vi "All parameter error estimate.vi"(8 "covariance":T2, 9 "best fit parameters":dbl[](array[numeric]), 10 "best nonlinear fit":dbl[](array[numeric]), 11 "Y":dbl[](array[numeric])) -> (0 "Status":i32[](array[numeric]), 1 "R-square":dbl, 2 "All FWHM":dbl[](array[numeric]), 3 "All Parameters Fit":T1(array[cluster]), 4 "List Status":string[][](table))   [LabVIEW 2023]
uses:
  <vilib>/Analysis/Matrix/Datatypes/RealMatrix.ctl
  <vilib>/Analysis/Matrix/Numeric/Conversions/Array To Matrix - RA2.vi
  <vilib>/Analysis/NI_AALPro.lvlib
  <vilib>/Analysis/Matrix/NI_Matrix.lvlib
panel:
  out "Correlation Matrix":T2
  out "Parameters Fit":T3
  out "FWHM":dbl
  out "Error":dbl[](array[numeric])
  out "RMSE":dbl
  out "SSE":dbl
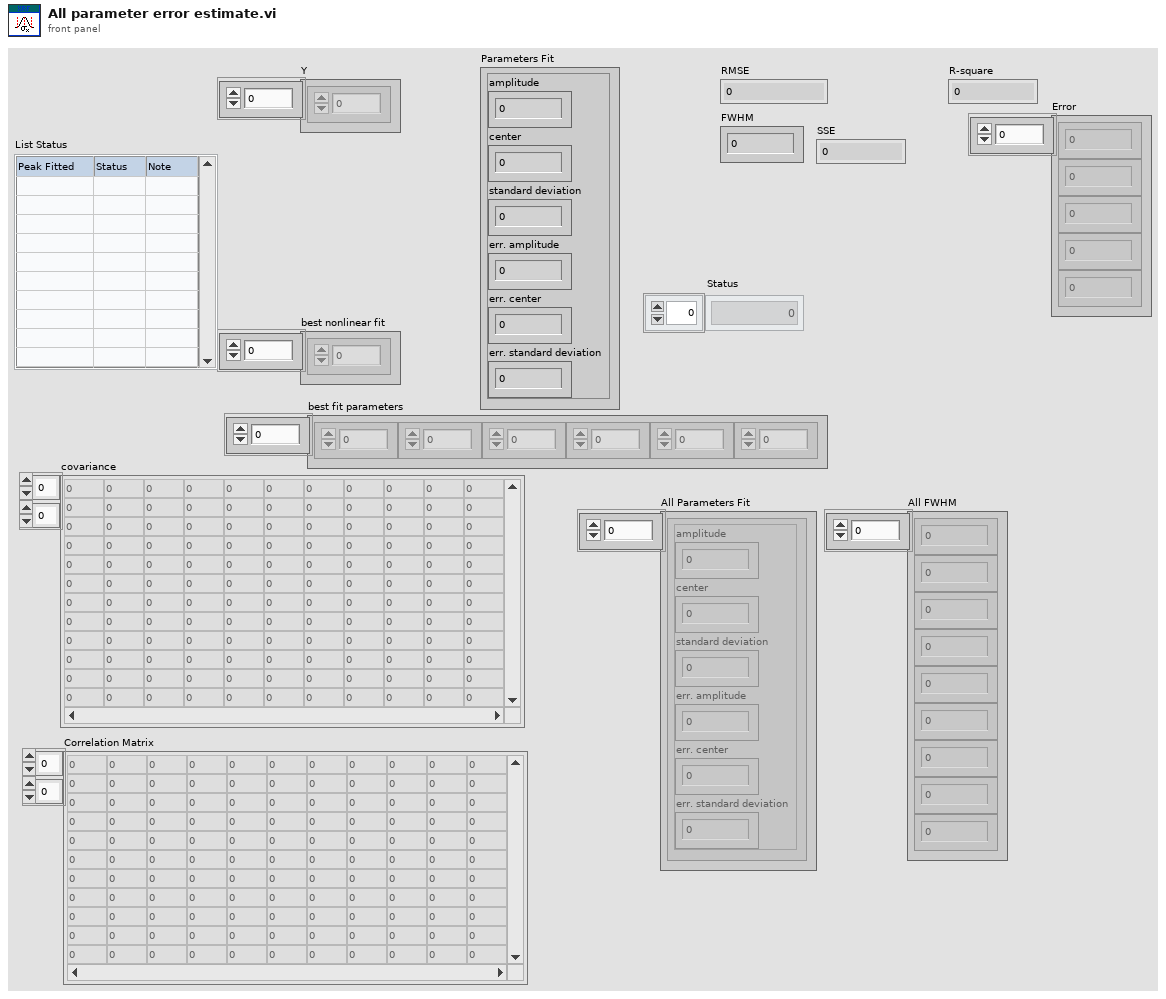
[diagram p1: front panel]
types:
  T1 = cluster{"amplitude":dbl, "center":dbl, "standard deviation":dbl, "err. amplitude":dbl, "err. center":dbl, "err. standard deviation":dbl}[]
  T2 = typedef "NI_Matrix.lvlib/RealMatrix.ctl" = dbl[][]
  T3 = cluster{"amplitude":dbl, "center":dbl, "standard deviation":dbl, "err. amplitude":dbl, "err. center":dbl, "err. standard deviation":dbl}
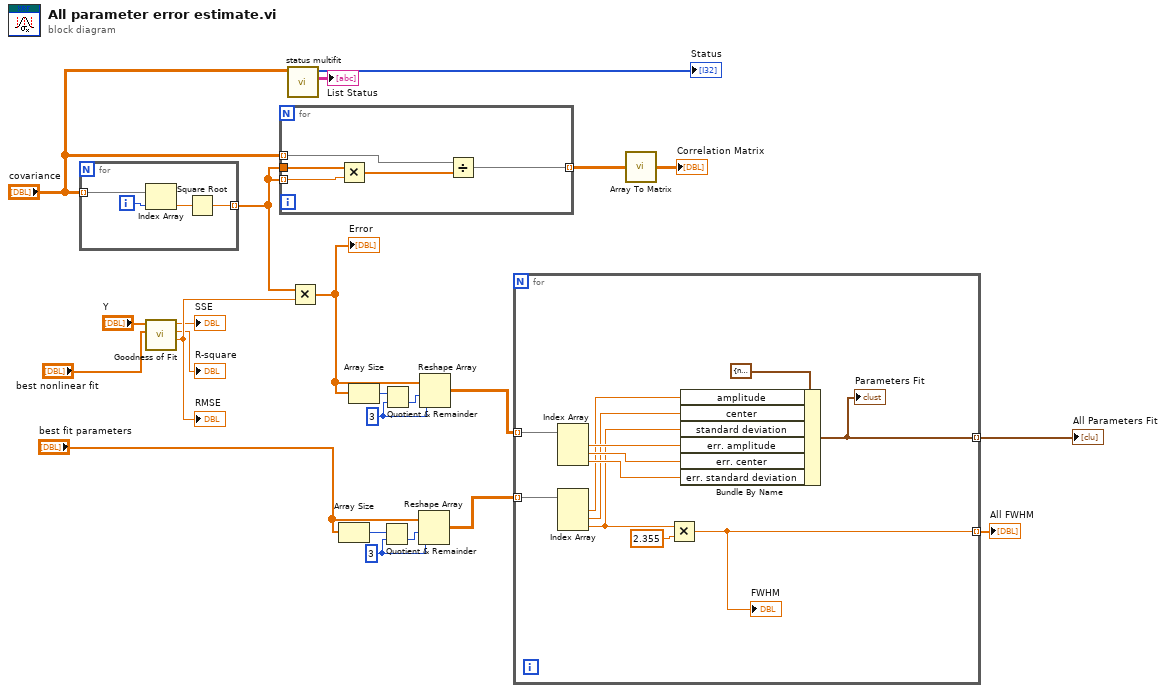
[diagram p0: block diagram]
diagram:
  w13 = 3 ("y")
  w14 = 3 ("y")
  n1 = for {
    tunnel: "covariance" -> [w27] mode=indexing
    tunnel: [w24] -> w19 mode=indexing
    i -> [w26]
    n2 = Index Array(array=w27, index=w26) -> (element=w25:dbl)
    n3 = Square Root(x=w25) -> (sqrt(x)=w24:dbl)
  }
  n4 = call <vilib>:"Goodness of Fit.vi"("Best Fit"="best nonlinear fit", "Y"="Y") -> ("RMSE"=w23:dbl, "R-square"=→"R-square":dbl, "SSE"=→"SSE":dbl)  [unwired: 6 in, 1 out]
  "RMSE" <- w23
  n5 = for {
    tunnel: "covariance" -> [w29] mode=indexing
    tunnel: w19 -> [w31]
    tunnel: w19 -> [w32] mode=indexing
    tunnel: [w28] -> w20 mode=indexing
    n6 = Multiply(x=w31, y=w32) -> (x*y=w30:dbl[])
    n7 = Divide(x=w29, y=w30) -> (x/y=w28:dbl[])
  }
  n8 = call "status multifit.vi"("covariance"="covariance") -> ("List Status"=→"List Status":string[][], "Status"=→"Status":i32[])  [unwired: 9 in]
  n9 = Multiply(x=w19, y=w23) -> (x*y=w8:dbl[])
  "Error" <- w8
  n10 = Array Size(array="best fit parameters") -> (size(s)=w7:i32)
  n11 = Array Size(array=w8) -> (size(s)=w9:i32)
  n12 = Quotient & Remainder(x=w7, y=w13) -> (floor(x/y)=w12:i32)  [unwired: 1 out]
  n13 = Quotient & Remainder(x=w9, y=w14) -> (floor(x/y)=w15:i32)  [unwired: 1 out]
  n14 = Reshape Array("best fit parameters", w12, w13) -> (w10:dbl[][])
  n15 = Reshape Array(w8, w15, w14) -> (w11:dbl[][])
  n16 = for {
    tunnel: w11 -> [w36] mode=indexing
    tunnel: w10 -> [w35] mode=indexing
    tunnel: [w34] -> w5 mode=indexing
    tunnel: [w33] -> w4 mode=indexing
    n17 = Index Array(array=w36) -> (element #1=w44:dbl, element #2=w43:dbl, element #3=w42:dbl)  [unwired: 3 in]
    n18 = Index Array(array=w35) -> (element #1=w39:dbl, element #2=w38:dbl, element #3=w41:dbl)  [unwired: 3 in]
    n19 = Multiply(x=w41, y=2.355) -> (x*y=w33:dbl)
    "FWHM" <- w33
    n20 = Bundle By Name(cluster=T3 {"amplitude"=nan, "center"=nan, "standard deviation"=nan, "err. amplitude"=nan, "err. center"=nan, "err. standard deviation"=nan} ("initial guess"), "amplitude"=w39, "center"=w38, "standard deviation"=w41, "err. amplitude"=w44, "err. center"=w43, "err. standard deviation"=w42) -> (w34:T3)
    "Parameters Fit" <- w34
  }
  "All Parameters Fit" <- w5
  "All FWHM" <- w4
  n21 = call-poly <vilib>:"Array To Matrix.vi"("Real 2D Array"=w20) -> ("Real Matrix"=→"Correlation Matrix":T2)
